vi "H5LTset_attribute_long.vi"(0 "error in (no error)":errorcluster, 2 "name":string, 6 "loc_id":i32, 7 "attr_name":string, 9 "buffer":i32[](array[numeric])) -> (3 "error out":errorcluster)   [LabVIEW 2009]
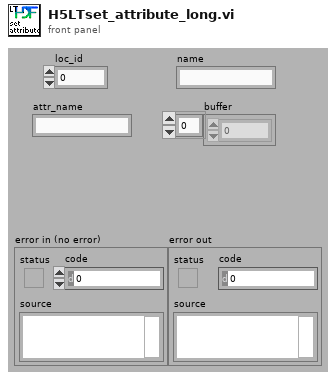
[diagram p1: front panel]
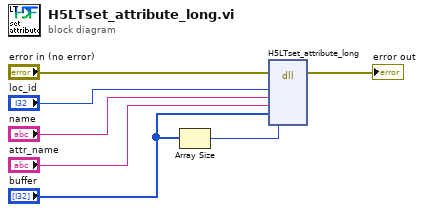
[diagram p0: block diagram]
diagram:
  n1 = Array Size(array="buffer") -> (size(s)=w1:i32)
  n2 = dll-call lib="hdf5_hldll" fn="H5LTset_attribute_long"(error in="error in (no error)", "loc_id"="loc_id", "name"="name", "attr_name"="attr_name", "buffer"="buffer", "size"=w1) -> (error out=→"error out":errorcluster)  [unwired: 8 in, 1 out]
